vi "LDO Load Transient - Flat.vi"(11 "error in (no error)":errorcluster) -> (15 "error out":errorcluster)   [LabVIEW 2020]
uses:
  <instrlib>/niScope/Controls/niScope vertical coupling.ctl
  <instrlib>/niScope/Controls/niScope trigger source digital.ctl
  <instrlib>/niDCPower/nidcpower.llb/niDCPower Output Function.ctl
  <instrlib>/niDCPower/nidcpower.llb/niDCPower Aperture Time Units.ctl
  <instrlib>/niDCPower/nidcpower.llb/niDCPower Source Mode.ctl
  <instrlib>/niDCPower/nidcpower.llb/niDCPower Export Signal - Signal.ctl
  <instrlib>/niDCPower/nidcpower.llb/niDCPower Wait For Event - Event.ctl
  <instrlib>/niScope/Controls/niScope trigger slope.ctl
  <instrlib>/niScope/Configure/Trigger/niScope Configure Trigger Digital.vi
  <instrlib>/niScope/Acquire/Fetch/niScope Multi Fetch Cluster.vi
  <instrlib>/niScope/Utility/niScope Get Channel Name From String.vi
  <vilib>/Utility/file.llb/Write Delimited Spreadsheet (DBL).vi
panel:
  in  "Tab Control":T1(tab)=enum."Test Parameters"
  in  "Scope":refnum<k15>="PXI1Slot5"
  in  "Source SMU":refnum<k15>="SMU1"
  in  "Load SMU":refnum<k15>="SMU1"
  in  "Source SMUCurrent Limit (A)":dbl=1.0
  in  "Source SMU Current Limit Range (A)":dbl=1.0
  in  "Source SMU Voltage Level Range (V)":dbl=8.0
  in  "Source SMU Channel":string="0"
  in  "Source Voltage (V)":dbl=6.0
  in  "Min. Record Length":i32=400000
  in  "Min. Sampling Rate":dbl=1000000.0
  in  "Trigger Modifier":i32(ring) items=["None", "Auto"]
  in  "Reference Position":dbl
  in  "Input Impedance":u32(ring) items=["1 Mega Ohm"=0, "50 Ohm"=2]
  in  "Trigger Delay (sec)":dbl
  in  "Max. Input Frequency (Hz)":dbl
  in  "Vertical Offset (V)":dbl
  in  "Probe Attentuation":dbl=1.0
  in  "Vertical Range (V)":dbl=5.0
  in  "Scope Channel":string="0"
  in  "Load SMU Voltage Limit (V)":dbl=8.0
  in  "Load SMU Transient Response":i32(ring)=1039 items=["Slow"=1041, "Normal"=1038, "Fast"=1039, "Custom"=1042]
  in  "Load SMU Record Length":i32=10
  in  "Load SMU Aperture Time (sec)":dbl=5e-06
  in  "Load SMU Voltage Limit Range (V)":dbl=8.0
  in  "Load SMU Current Level Range (A)":dbl=1.0
  in  "Load SMU Channel":string="1"
  in  "Load  SMU Current Level (A)":dbl=-0.05
  in  "Vertical Coupling":T2 items=["AC", "DC", "Ground"]
  in  "Trigger Source":T3="VAL_PFI_0" caption="trigger source (RTSI 0)"
  out "Settling Time (s)":dbl format="%#_6p"
  in  "Recovery Level (V)":dbl=0.01
  in  "Iload2 Current Level Width (sec)":dbl=0.1
  in  "Load Current 2 - Iload 2":dbl=-0.15
  in  "Load Current 1 - Iload 1":dbl=-0.05
  out "Mixed Signal Graph":cluster{waveform(dbl), waveform(dbl)}(graph)={{"t0"=timestamp(0 s since 1904-01-01), "dt"=4.9999999999999996e-06, "Y"=array[60000 elements]}, {"t0"=timestamp(0 s since 1904-01-01), "dt"=4.9999999999999996e-06, "Y"=array[60000 elements]}}
  out "Waveform Graph":T4(graph)
  out "Waveform(s)":T5(graph)={"relativeInitialX"=1e-06, "xIncrement"=1e-06, "wfm"=array[300000 elements]} caption="Instantaneous Load Transient Waveform"
  # "Load Transient Measurement - Flat VI"
  # "Load SMU Config"
  # "Source SMU Config"
  # "Scope Config"
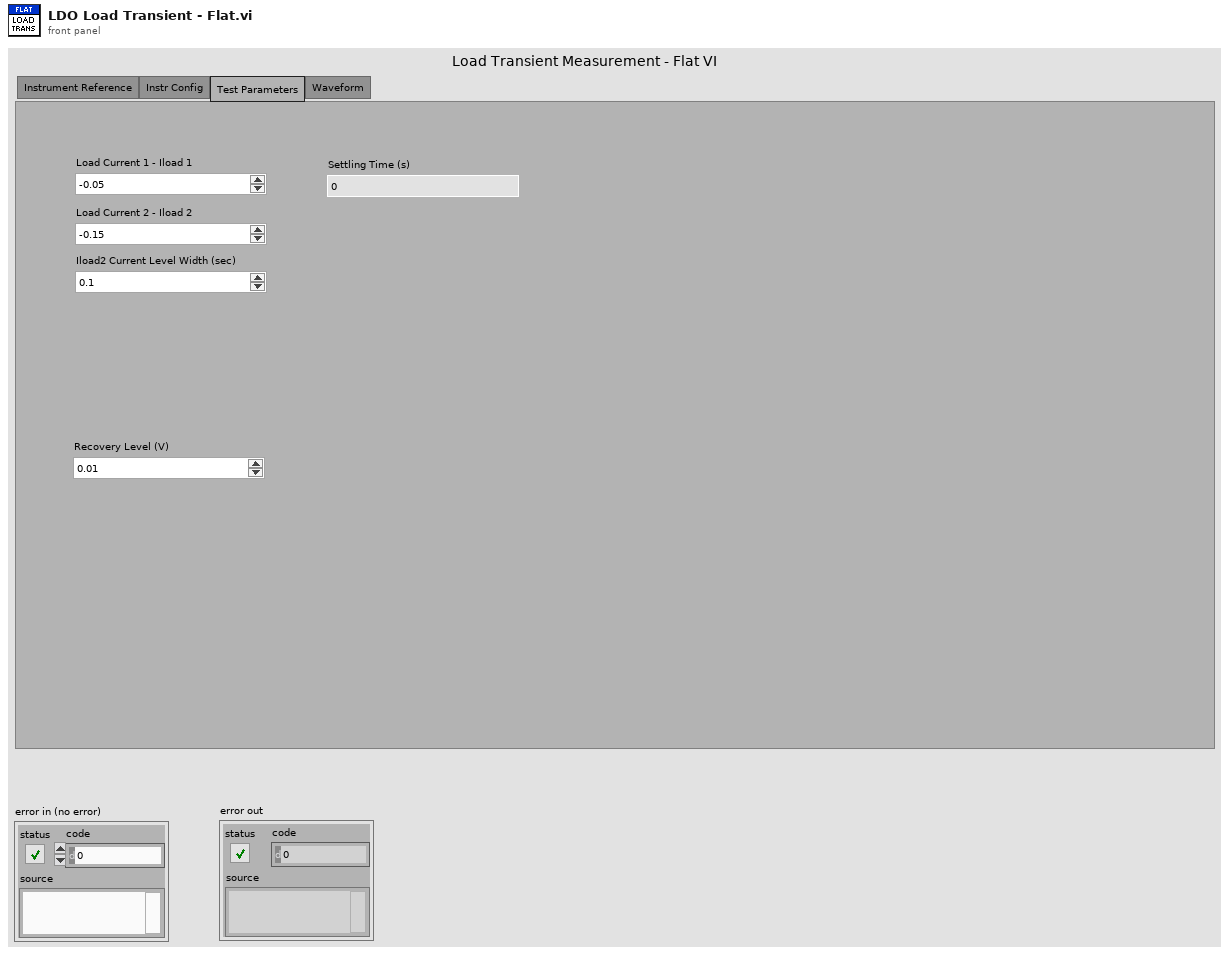
[diagram p1: front panel]
types:
  T1 = enum32{"Instrument Reference", "Instr Config", "Test Parameters", "Waveform"}
  T2 = typedef "niScope vertical coupling.ctl" = i32
  T3 = typedef "niScope trigger source digital.ctl" = string
  T4 = cluster{dbl, "Measure Record dt":dbl, "voltage measurements":dbl[]}
  T5 = cluster{"relativeInitialX":dbl, "xIncrement":dbl, "wfm":dbl[]}
  T6 = typedef "niDCPower Output Function.ctl" = i32
  T7 = typedef "niDCPower Source Mode.ctl" = i32
  T8 = typedef "niScope trigger slope.ctl" = i32
  T9 = typedef "niDCPower Wait For Event - Event.ctl" = i32
  T10 = typedef "niDCPower Export Signal - Signal.ctl" = i32
  T11 = typedef "niDCPower Aperture Time Units.ctl" = i32
  T12 = cluster{"relativeInitialX":dbl, "xIncrement":dbl, "wfm":dbl[]}[]
  T13 = cluster{dbl, "Measure Record dt":dbl, "current measurements":dbl[]}
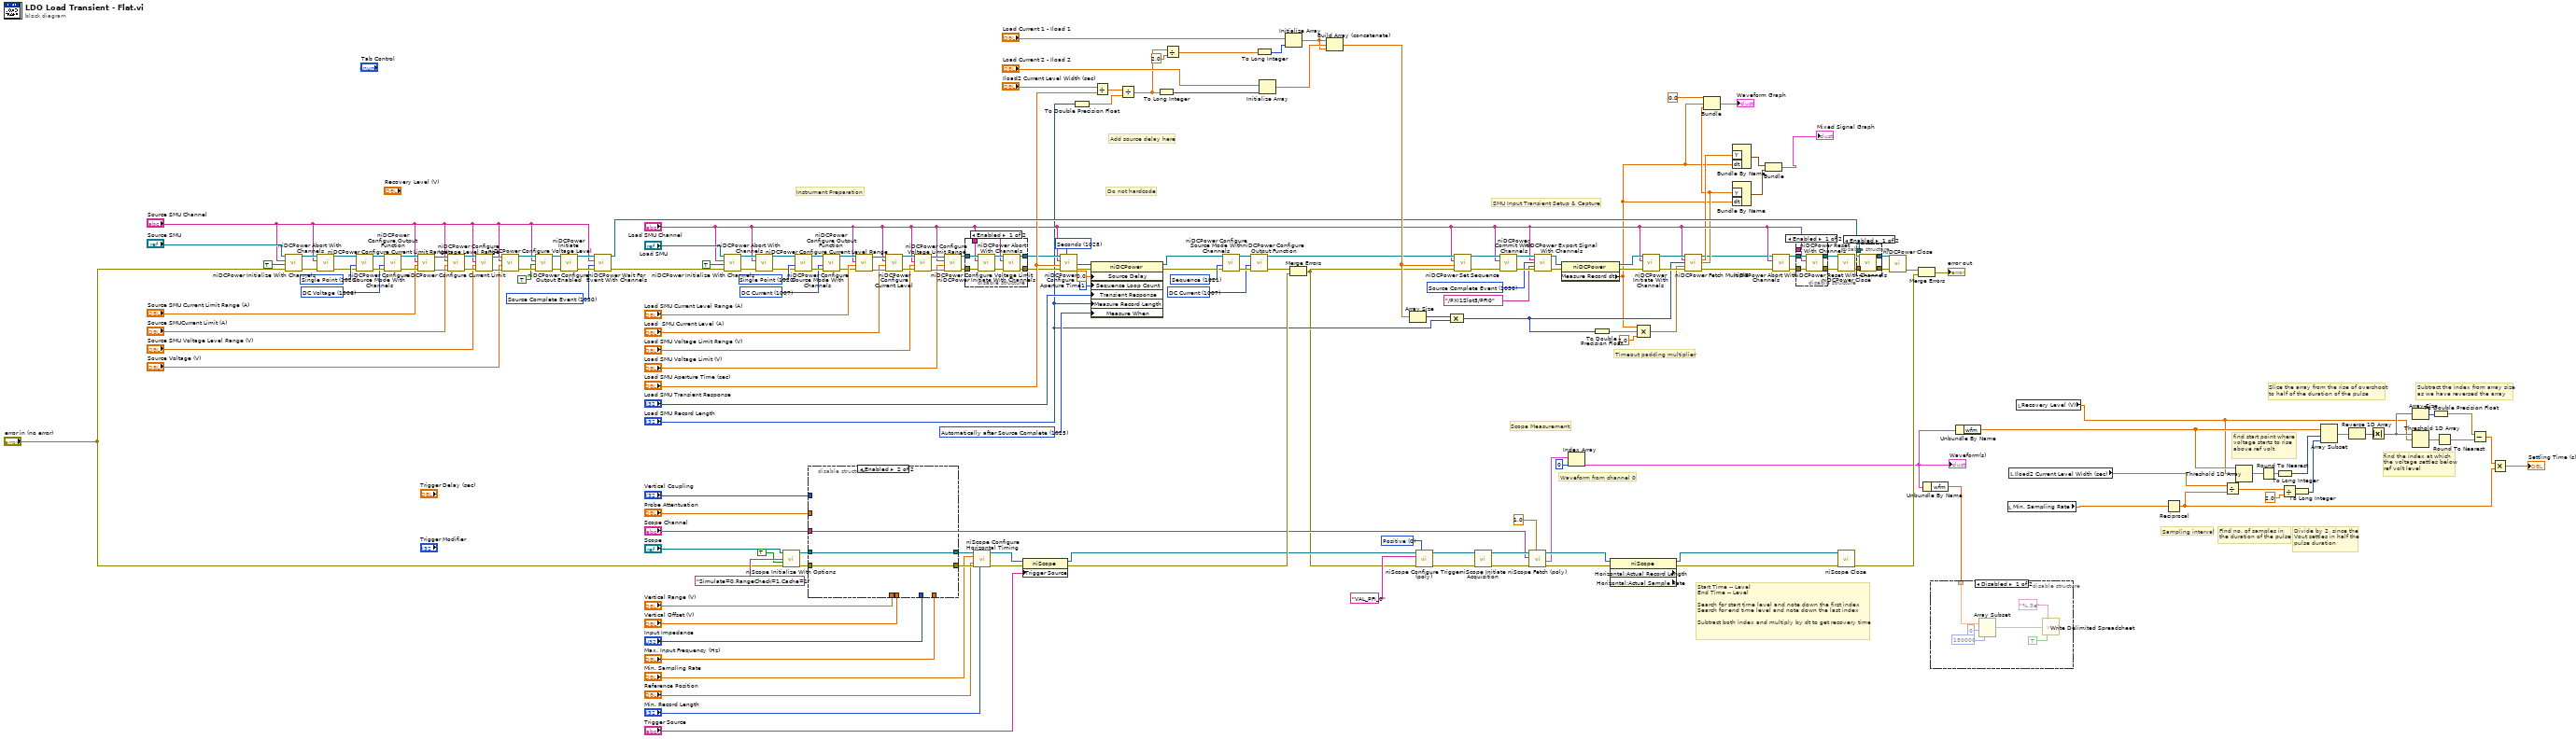
[diagram p0: block diagram]
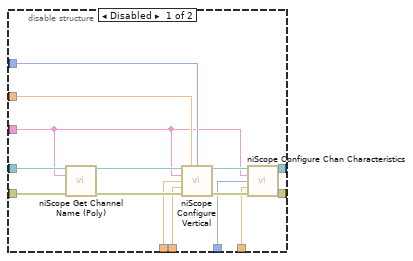
[diagram p2: hidden frame]
diagram:
  w52 = T6 1007 items=["DC Voltage"=1006, "DC Current"=1007, "Pulse Voltage"=1049, "Pulse Current"=1050] ("output function")
  w53 = T7 1021 items=["Single Point"=1020, "Sequence"=1021] ("source mode")
  w41 = T8 0 items=["Positive", "Negative"] ("trigger slope")
  w77 = T9 1030 items=["Source Complete Event"=1030, "Measure Complete Event"=1031, "Sequence Iteration Complete Event"=1032, "Sequence Engine Done Event"=1033, "Pulse Complete Event"=1051, "Ready For Pulse Trigger Event"=1052] ("event")
  w107 = T10 1030 items=["Source Complete Event"=1030, "Measure Complete Event"=1031, "Sequence Iteration Complete Event"=1032, "Sequence Engine Done Event"=1033, "Pulse Complete Event"=1051, "Ready For Pulse Trigger Event"=1052, "Start Trigger"=1034, "Source Trigger"=1035, "Measure Trigger"=1036, "Sequence Advance Trigger"=1037, "Pulse Trigger"=1053] ("signal")
  w152 = T6 1006 items=["DC Voltage"=1006, "DC Current"=1007, "Pulse Voltage"=1049, "Pulse Current"=1050] ("output function")
  w153 = T7 1020 items=["Single Point"=1020, "Sequence"=1021] ("source mode")
  w161 = 1025 items=["Automatically after Source Complete"=1025, "On Demand"=1026, "On Measure Trigger"=1027] ("Measurement:Advanced:Measure When")
  w169 = T11 1028 items=["Seconds"=1028, "Powerline Cycles"=1029] ("aperture time units")
  w172 = T6 1007 items=["DC Voltage"=1006, "DC Current"=1007, "Pulse Voltage"=1049, "Pulse Current"=1050] ("output function")
  w173 = T7 1020 items=["Single Point"=1020, "Sequence"=1021] ("source mode")
  # "Subtract the index from array size\nas we have reversed the array"
  # "Sampling interval"
  # "find the index at which \nthe voltage settles below\nref volt level"
  # "Slice the array from the rise of overshoot\nto half of the duration of the pulse"
  # "Divide by 2, since the\nVout settles in half the\npulse duration"
  # "Find no. of samples in \nthe duration of the pulse"
  # "find start point where voltage starts to rise above ref volt"
  # "Add source delay here"
  # "Do not hardcode"
  # "Start Time -- Level\nEnd Time -- Level\n\nSearch for start time level and note down the first index\nSearch for end time level and note down the last index\n\nSubtract both index and multiply by dt to get recovery time"
  # "SMU Input Transient Setup & Capture"
  # "Scope Measurement"
  # "Waveform from channel 0"
  # "Timeout padding multiplier"
  # "Instrument Preparation"
  n1 = call <instrlib>:"niDCPower Initialize With Channels.vi"("error in (no error)"="error in (no error)", "reset (false)"=TRUE, "channels"="Source SMU Channel", "resource name"="Source SMU") -> ("error out"=w149:errorcluster, "instrument handle out"=w147:refnum<k15>)  [unwired: 1 in, 5 out]
  n2 = call <instrlib>:"niDCPower Abort With Channels.vi"("error in (no error)"=w149, "channel name"="Source SMU Channel", "instrument handle"=w147) -> ("error out"=w148:errorcluster, "instrument handle out"=w146:refnum<k15>)  [unwired: 7 in]
  n3 = call <instrlib>:"niDCPower Configure Source Mode With Channels.vi"("error in (no error)"=w148, "source mode"=w153, "instrument handle"=w146) -> ("error out"=w154:errorcluster, "instrument handle out"=w155:refnum<k15>)  [unwired: 7 in]
  n4 = call <instrlib>:"niDCPower Configure Output Function.vi"("error in (no error)"=w154, "output function"=w152, "instrument handle"=w155) -> ("error out"=w150:errorcluster, "instrument handle out"=w151:refnum<k15>)  [unwired: 7 in]
  n5 = call <instrlib>:"niDCPower Configure Current Limit Range.vi"("error in (no error)"=w150, "current limit range"="Source SMU Current Limit Range (A)", "channel name"="Source SMU Channel", "instrument handle"=w151) -> ("error out"=w160:errorcluster, "instrument handle out"=w159:refnum<k15>)  [unwired: 6 in]
  n6 = call <instrlib>:"niDCPower Configure Current Limit.vi"("error in (no error)"=w160, "current limit"="Source SMUCurrent Limit (A)", "channel name"="Source SMU Channel", "instrument handle"=w159) -> ("error out"=w158:errorcluster, "instrument handle out"=w157:refnum<k15>)  [unwired: 6 in]
  n7 = call <instrlib>:"niDCPower Configure Voltage Level Range.vi"("error in (no error)"=w158, "voltage level range"="Source SMU Voltage Level Range (V)", "channel name"="Source SMU Channel", "instrument handle"=w157) -> ("error out"=w143:errorcluster, "instrument handle out"=w144:refnum<k15>)  [unwired: 6 in]
  n8 = call <instrlib>:"niDCPower Configure Voltage Level.vi"("error in (no error)"=w143, "voltage level"="Source Voltage (V)", "channel name"="Source SMU Channel", "instrument handle"=w144) -> ("error out"=w82:errorcluster, "instrument handle out"=w79:refnum<k15>)  [unwired: 6 in]
  n9 = call <instrlib>:"niDCPower Configure Output Enabled.vi"("error in (no error)"=w82, "output enabled"=TRUE, "channel name"="Source SMU Channel", "instrument handle"=w79) -> ("error out"=w81:errorcluster, "instrument handle out"=w84:refnum<k15>)  [unwired: 6 in]
  n10 = call <instrlib>:"niDCPower Initiate.vi"("error in (no error)"=w81, "instrument handle"=w84) -> ("error out"=w80:errorcluster, "instrument handle out"=w83:refnum<k15>)  [unwired: 8 in]
  n11 = call <instrlib>:"niDCPower Wait For Event With Channels.vi"("error in (no error)"=w80, "event"=w77, "channel name"="Source SMU Channel", "instrument handle"=w83) -> ("error out"=w34:errorcluster, "instrument handle out"=w59:refnum<k15>)  [unwired: 6 in]
  n12 = call <instrlib>:"niDCPower Initialize With Channels.vi"("error in (no error)"=w34, "reset (false)"=TRUE, "channels"="Load SMU Channel", "resource name"="Load SMU") -> ("error out"=w168:errorcluster, "instrument handle out"=w166:refnum<k15>)  [unwired: 1 in, 5 out]
  n13 = call <instrlib>:"niDCPower Abort With Channels.vi"("error in (no error)"=w168, "channel name"="Load SMU Channel", "instrument handle"=w166) -> ("error out"=w167:errorcluster, "instrument handle out"=w165:refnum<k15>)  [unwired: 7 in]
  n14 = call <instrlib>:"niScope Initialize With Options.vi"("resource name"="Scope", "option string"="Simulate=0,RangeCheck=1,Cache=1", "reset device"=TRUE, "error in"="error in (no error)") -> ("instrument handle"=w138:refnum<k15>, "error out"=w137:errorcluster)  [unwired: 10 in]
  n15 = call <instrlib>:"niDCPower Configure Source Mode With Channels.vi"("error in (no error)"=w167, "source mode"=w173, "instrument handle"=w165) -> ("error out"=w174:errorcluster, "instrument handle out"=w175:refnum<k15>)  [unwired: 7 in]
  n16 = disable-structure shown="Enabled" {
    disable-tunnel: w138 -> [w202 w203]
    disable-tunnel: w137 -> [w201 w204]
    disable-tunnel: [w198 w204] -> w136
    disable-tunnel: [w197 w203] -> w135
    disable-tunnel: "Probe Attentuation" -> [w194 _]
    disable-tunnel: "Vertical Coupling" -> [w193 _]
    disable-tunnel: "Vertical Range (V)" -> [w192 _]
    disable-tunnel: "Vertical Offset (V)" -> [w191 _]
    disable-tunnel: "Max. Input Frequency (Hz)" -> [w190 _]
    disable-tunnel: "Input Impedance" -> [w189 _]
    disable-tunnel: "Scope Channel" -> [w188 _]
    frame Disabled {
      n17 = call-poly <instrlib>:"niScope Get Channel Name (Poly).vi"("instrument handle"=w202, "index"=w188, "error in"=w201) -> ("instrument handle out"=w196:refnum<k15>, "error out"=w195:errorcluster)  [unwired: 10 in, 1 out]
      n18 = call <instrlib>:"niScope Configure Vertical.vi"("instrument handle"=w196, "probe attenuation"=w194, "vertical coupling"=w193, "channels"=w188, "vertical range"=w192, "vertical offset"=w191, "error in"=w195) -> ("instrument handle out"=w200:refnum<k15>, "error out"=w199:errorcluster)  [unwired: 7 in]
      n19 = call <instrlib>:"niScope Configure Chan Characteristics.vi"("instrument handle"=w200, "channels"=w188, "input impedance"=w189, "maximum input frequency"=w190, "error in"=w199) -> ("instrument handle out"=w197:refnum<k15>, "error out"=w198:errorcluster)  [unwired: 9 in]
    }
    frame Enabled {
    }
  }
  n20 = call <instrlib>:"niDCPower Configure Output Function.vi"("error in (no error)"=w174, "output function"=w172, "instrument handle"=w175) -> ("error out"=w170:errorcluster, "instrument handle out"=w171:refnum<k15>)  [unwired: 7 in]
  n21 = call <instrlib>:"niDCPower Configure Current Level Range.vi"("error in (no error)"=w170, "current level range"="Load SMU Current Level Range (A)", "channel name"="Load SMU Channel", "instrument handle"=w171) -> ("error out"=w187:errorcluster, "instrument handle out"=w186:refnum<k15>)  [unwired: 6 in]
  n22 = call <instrlib>:"niDCPower Configure Current Level.vi"("error in (no error)"=w187, "current level"="Load  SMU Current Level (A)", "channel name"="Load SMU Channel", "instrument handle"=w186) -> ("error out"=w185:errorcluster, "instrument handle out"=w184:refnum<k15>)  [unwired: 6 in]
  n23 = call <instrlib>:"niDCPower Configure Voltage Limit Range.vi"("error in (no error)"=w185, "voltage limit range"="Load SMU Voltage Limit Range (V)", "channel name"="Load SMU Channel", "instrument handle"=w184) -> ("error out"=w183:errorcluster, "instrument handle out"=w182:refnum<k15>)  [unwired: 6 in]
  n24 = call <instrlib>:"niDCPower Configure Voltage Limit.vi"("error in (no error)"=w183, "voltage limit"="Load SMU Voltage Limit (V)", "channel name"="Load SMU Channel", "instrument handle"=w182) -> ("error out"=w46:errorcluster, "instrument handle out"=w44:refnum<k15>)  [unwired: 6 in]
  n25 = disable-structure shown="Enabled" {
    disable-tunnel: w46 -> [w209 w212]
    disable-tunnel: [w208 w212] -> w45
    disable-tunnel: w44 -> [w207 w213]
    disable-tunnel: [w206 w213] -> w43
    disable-tunnel: "Load SMU Channel" -> [w205 _]
    frame Enabled {
      n26 = call <instrlib>:"niDCPower Initiate With Channels.vi"("error in (no error)"=w209, "channel name"=w205, "instrument handle"=w207) -> ("error out"=w211:errorcluster, "instrument handle out"=w210:refnum<k15>)  [unwired: 7 in]
      n27 = call <instrlib>:"niDCPower Abort With Channels.vi"("error in (no error)"=w211, "channel name"=w205, "instrument handle"=w210) -> ("error out"=w208:errorcluster, "instrument handle out"=w206:refnum<k15>)  [unwired: 7 in]
    }
    frame Disabled {
    }
  }
  n28 = call <instrlib>:"niScope Configure Horizontal Timing.vi"("instrument handle"=w135, "min sample rate"="Min. Sampling Rate", "reference position"="Reference Position", "error in"=w136, "min record length"="Min. Record Length") -> ("instrument handle out"=w121:refnum<k15>, "error out"=w122:errorcluster)  [unwired: 9 in]
  n29 = property class="niScope"(reference=w121, error in=w122, "Trigger Source"="Trigger Source") -> (reference out=w73:refnum<k15>, error out=w75:errorcluster)
  n30 = call <instrlib>:"niDCPower Configure Aperture Time.vi"("aperture time units"=w169, "error in (no error)"=w45, "aperture time"="Load SMU Aperture Time (sec)", "channel name"="Load SMU Channel", "instrument handle"=w43) -> ("error out"=w85:errorcluster, "instrument handle out"=w39:refnum<k15>)  [unwired: 5 out]
  n31 = To Double Precision Float(number="Load SMU Record Length") -> (double precision float=w36:dbl)
  n32 = property class="niDCPower"(reference=w39, error in=w85, "Source Delay"=0.0 ("Source:Advanced:Source Delay"), "Sequence Loop Count"=1 ("Source:Advanced:Sequence Loop Count"), "Transient Response"="Load SMU Transient Response", "Measure Record Length"="Load SMU Record Length", "Measure When"=w161) -> (reference out=w48:refnum<k15>, error out=w51:errorcluster)
  n33 = Divide(x="Iload2 Current Level Width (sec)", y="Load SMU Aperture Time (sec)") -> (x/y=w38:dbl)
  n34 = Divide(x=w38, y=w36) -> (x/y=w35:dbl)
  n35 = To Long Integer(number=w35) -> (32bit integer=w119:i32)
  n36 = Divide(x=w35, y=2.0) -> (x/y=w115:dbl)
  n37 = call <instrlib>:"niDCPower Configure Source Mode With Channels.vi"("error in (no error)"=w51, "source mode"=w53, "instrument handle"=w48) -> ("error out"=w54:errorcluster, "instrument handle out"=w49:refnum<k15>)  [unwired: 7 in]
  n38 = call <instrlib>:"niDCPower Configure Output Function.vi"("error in (no error)"=w54, "output function"=w52, "instrument handle"=w49) -> ("error out"=w50:errorcluster, "instrument handle out"=w47:refnum<k15>)  [unwired: 7 in]
  n39 = To Long Integer(number=w115) -> (32bit integer=w114:i32)
  n40 = Initialize Array("Load Current 2 - Iload 2", w119) -> (w113:dbl[])
  n41 = Initialize Array("Load Current 1 - Iload 1", w114) -> (w112:dbl[])
  n42 = Merge Errors(w50, w75) -> (w33:errorcluster)
  n43 = Build Array (concatenate)(w112, w113, w112) -> (w103:dbl[])
  n44 = Array Size(array=w103) -> (size(s)=w102:i32)
  n45 = call-poly <instrlib>:"niScope Configure Trigger (poly).vi"("instrument handle"=w73, "trigger slope"=w41, "trigger source"=T3 "VAL_PFI_0", "error in"=w33) -> ("instrument handle out"=w74:refnum<k15>, "error out"=w87:errorcluster)  [unwired: 10 in]
  n46 = Compound Arithmetic op=MULTIPLY(w102, "Load SMU Record Length") -> (w95:i32)
  n47 = call <instrlib>:"niDCPower Set Sequence.vi"("error in (no error)"=w33, "values"=w103, "channel name"="Load SMU Channel", "instrument handle"=w47) -> ("error out"=w111:errorcluster, "instrument handle out"=w110:refnum<k15>)  [unwired: 1 in, 5 out]
  n48 = call <instrlib>:"niScope Initiate Acquisition.vi"("instrument handle"=w74, "error in"=w87) -> ("instrument handle out"=w71:refnum<k15>, "error out"=w86:errorcluster)  [unwired: 12 in]
  n49 = call <instrlib>:"niDCPower Commit With Channels.vi"("error in (no error)"=w111, "channel name"="Load SMU Channel", "instrument handle"=w110) -> ("error out"=w109:errorcluster, "instrument handle out"=w108:refnum<k15>)  [unwired: 7 in]
  n50 = call-poly <instrlib>:"niScope Fetch (poly).vi"("timeout"=1.0, "error in"=w86, "channels"="Scope Channel", "instrument handle"=w71) -> ("error out"=w88:errorcluster, "waveform"=w67:T12, "instrument handle out"=w68:refnum<k15>)  [unwired: 4 in, 1 out]
  n51 = call <instrlib>:"niDCPower Export Signal With Channels.vi"("instrument handle"=w108, "channel name"="Load SMU Channel", "signal"=w107, "output terminal"=tag "/PXI1Slot5/PFI0", "error in (no error)"=w109) -> ("instrument handle out"=w104:refnum<k15>, "error out"=w105:errorcluster)  [unwired: 9 in]
  n52 = property class="niDCPower"(reference=w104, error in=w105) -> (reference out=w98:refnum<k15>, error out=w99:errorcluster, "Measure Record dt"=w26:dbl)
  n53 = Index Array(array=w67, index=0) -> (element=w4:T5)
  "Waveform(s)" <- w4
  n54 = To Double Precision Float(number=w95) -> (double precision float=w100:dbl)
  n55 = property class="niScope" props=["Horizontal:Actual Record Length", "Horizontal:Actual Sample Rate"](reference=w68, error in=w88) -> (reference out=w64:refnum<k15>, error out=w65:errorcluster)  [unwired: 2 out]
  n56 = Compound Arithmetic op=MULTIPLY(w26, w100, 2.0 ("value")) -> (w94:dbl)
  n57 = call <instrlib>:"niDCPower Initiate With Channels.vi"("error in (no error)"=w99, "channel name"="Load SMU Channel", "instrument handle"=w98) -> ("error out"=w97:errorcluster, "instrument handle out"=w96:refnum<k15>)  [unwired: 7 in]
  n58 = call <instrlib>:"niDCPower Fetch Multiple.vi"("instrument handle"=w96, "channel name"="Load SMU Channel", "count (1)"=w95, "timeout (sec)"=w94, "error in (no error)"=w97) -> ("instrument handle out"=w24:refnum<k15>, "voltage measurements"=w29:dbl[], "current measurements"=w27:dbl[], "error out"=w25:errorcluster)  [unwired: 7 out]
  n59 = Bundle(0.0, "Measure Record dt"=w26, "current measurements"=w27) -> (→"Waveform Graph":T13)  [unwired: 1 in]
  n60 = Bundle By Name("Y"=w29, "dt"=w26) -> (w89:waveform(dbl))  [unwired: 1 out]
  n61 = Bundle By Name("Y"=w27, "dt"=w26) -> (w56:waveform(dbl))  [unwired: 1 out]
  n62 = Bundle(w89, w56) -> (→"Mixed Signal Graph":cluster{waveform(dbl), waveform(dbl)})  [unwired: 1 in]
  n63 = call <instrlib>:"niDCPower Abort With Channels.vi"("error in (no error)"=w25, "channel name"="Load SMU Channel", "instrument handle"=w24) -> ("error out"=w92:errorcluster, "instrument handle out"=w90:refnum<k15>)  [unwired: 7 in]
  n64 = disable-structure shown="Enabled" {
    disable-tunnel: [w218 w220] -> w93
    disable-tunnel: w92 -> [w217 w219]
    disable-tunnel: [w216 w219] -> w91
    disable-tunnel: w90 -> [w215 w220]
    disable-tunnel: "Load SMU Channel" -> [w214 _]
    frame Enabled {
      n65 = call <instrlib>:"niDCPower Reset With Channels.vi"("error in (no error)"=w217, "channel name"=w214, "instrument handle"=w215) -> ("error out"=w216:errorcluster, "instrument handle out"=w218:refnum<k15>)  [unwired: 7 in]
    }
    frame Disabled {
    }
  }
  n66 = call <instrlib>:"niDCPower Close.vi"("error in (no error)"=w91, "instrument handle"=w93) -> ("error out"=w32:errorcluster)  [unwired: 9 out]
  n67 = call <instrlib>:"niScope Close.vi"("instrument handle"=w64, "error in"=w65) -> ("error out"=w63:errorcluster)  [unwired: 13 in]
  n68 = disable-structure shown="Enabled" {
    disable-tunnel: [w224 w226] -> w61
    disable-tunnel: [w223 w225] -> w60
    disable-tunnel: w59 -> [w222 w226]
    disable-tunnel: w32 -> [w221 w225]
    frame Enabled {
      n69 = call <instrlib>:"niDCPower Reset With Channels.vi"("error in (no error)"=w221, "instrument handle"=w222) -> ("error out"=w223:errorcluster, "instrument handle out"=w224:refnum<k15>)  [unwired: 8 in]
    }
    frame Disabled {
    }
  }
  n70 = call <instrlib>:"niDCPower Close.vi"("error in (no error)"=w60, "instrument handle"=w61) -> ("error out"=w31:errorcluster)  [unwired: 9 out]
  n71 = Merge Errors(w31, w63) -> (→"error out":errorcluster)
  n72 = Unbundle By Name(w4) -> ("wfm"=w23:dbl[])
  n73 = disable-structure shown="Disabled" {
    disable-tunnel: w23 -> [w232 _]
    frame Disabled {
      n74 = Array Subset(array=w232, index=0, length=150000) -> (w229:dbl[])
      n75 = call-poly <vilib>:"Write Delimited Spreadsheet.vi"("format (%.3f)"="%.3e", "1D data"=w229, "transpose? (no:F)"=TRUE) -> ()  [unwired: 11 in, 2 out]
    }
    frame Enabled {
    }
  }
  n76 = Unbundle By Name(w4) -> ("wfm"=w3:dbl[])
  n77 = local read "Min. Sampling Rate"() -> (w6:dbl)
  n78 = local read "Iload2 Current Level Width (sec)"() -> (w5:dbl)
  n79 = local read "Recovery Level (V)"() -> (w2:dbl)
  n80 = Reciprocal(x=w6) -> (1/x=w14:dbl)
  n81 = Divide(x=w5, y=w14) -> (x/y=w20:dbl)
  n82 = Threshold 1D Array(2:w2, 3:w3) -> (0:w22:dbl)  [unwired: 1 in]
  n83 = Round To Nearest(number=w22) -> (nearest integer value=w21:dbl)
  n84 = To Long Integer(number=w21) -> (32bit integer=w13:i32)
  n85 = Divide(x=w20, y=2.0) -> (x/y=w18:dbl)
  n86 = To Long Integer(number=w18) -> (32bit integer=w17:i32)
  n87 = Array Subset(array=w3, index=w13, length=w17) -> (w12:dbl[])
  n88 = Reverse 1D Array(array=w12) -> (reversed array=w16:dbl[])
  n89 = Absolute Value(x=w16) -> (abs(x)=w9:dbl[])
  n90 = Threshold 1D Array(2:w2, 3:w9) -> (0:w15:dbl)  [unwired: 1 in]
  n91 = Array Size(array=w9) -> (size(s)=w8:i32)
  n92 = To Double Precision Float(number=w8) -> (double precision float=w7:dbl)
  n93 = Round To Nearest(number=w15) -> (nearest integer value=w11:dbl)
  n94 = Subtract(x=w7, y=w11) -> (x-y=w10:dbl)
  n95 = Multiply(x=w10, y=w14) -> (x*y=→"Settling Time (s)":dbl)
